vi "test_ccd_parseImageData.vi"(8 "error in (no error)":errorcluster) -> (0 "error out":errorcluster)   [LabVIEW 2023, in "horiba.test.lvlib"]
uses:
  horiba.test.lvlib
  Classes/CCD/acquisitionData.ctl
  Classes/CCD/CCDImageData.ctl
  <vilib>/addons/_JKI Toolkits/Caraya/classes/Assert/Assert Not Error.vi
  <vilib>/addons/_JKI Toolkits/Caraya/classes/Assert/Assert Equal Value and Type_Variant.vi
  <vilib>/addons/_JKI Toolkits/Caraya/classes/Test/Test.lvclass
  <vilib>/addons/_JKI Toolkits/Caraya/classes/Assert/Assert.lvclass
  Classes/CCD/CCD.lvclass
panel:
  # "Connector Pane"
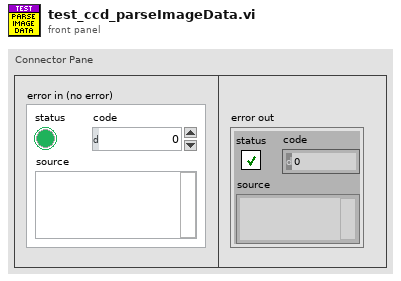
[diagram p1: front panel]
types:
  T1 = typedef "horiba.lvlib/CCD.lvclass/acquisitionData.ctl" = cluster{"acqIndex":i32, "ROIs":T2[]}
  T2 = typedef "horiba.lvlib/CCD.lvclass/CCDImageData.ctl" = cluster{"roiIndex":i32, "xBinning":i32, "xOrigin":i32, "xSize":i32, "yBinning":i32, "yOrigin":i32, "ySize":i32, "xAxis":dbl[], "Data":dbl[][]}
  T3 = typedef "acquisitionData.ctl" = cluster{"acqIndex":i32, "ROIs":T2[]}
diagram:
  n1 = call <vilib>:"Define Test.vi"("error in (no error)"="error in (no error)") -> ("error out"=w7:errorcluster)  [unwired: 9 in, 1 out]
  "error out" <- w7
  n2 = call "parseImageData.vi"("results-JSON string"="{\"acquisition\":[{\"acqIndex\":1,\"roi\":[{\"roiIndex\":1,\"xBinning\":1,\"xOrigin\":0,\"xSize\":1024,\"xyData\":[[0,608],[1,606],[2,607],[3,606],[4,605],[5,606],[6,604],[7,607],[8,605],[9,605],[10,606],[11,606],[12,604],[13,604],[14,604],[15,607],[16,606],[17,606],[18,604],[19,606],[20,607],[21,607],[22,606],[23,608],[24,606],[25,605],[26,607],[27,605],[28,607],[29,607],[30,604],[31,606],[32,608],[33,605],[34,606],[35,607],[36,603],[37,605],[38,605],[39,606],[40,605],[41,606],[42,605],[43,607],[44,606],[45,607],[46,605],[47,605],[48,607],[49,606],[50,606],[51,606],[52,605],[53,607],[54,607],[55,604],[56,607],[57,608],[58,607],[59,608],[60,606],[61,605],[62,608],[63,606],[64,605],[65,606],[66,604],[67,607],[68,607],[69,607],[70,611],[71,608],[72,606],[73,608],[74,607],[75,603],[76,604],[77,607],[78,604],[79,606],[80,606],[81,608],[82,603],[83,604],[84,607],[85,605],[86,605],[87,605],[88,607],[89,605],[90,606],[91,606],[92,608],[93,605],[94,606],[95,605],[96,609],[97,606],[98,609],[99,606],[100,605],[101,605],[102,607],[103,605],[104,606],[105,605],[106,607],[107,605],[108,607],[109,609],[110,604],[111,605],[112,605],[113,606],[114,606],[115,604],[116,606],[117,608],[118,606],[119,606],[120,603],[121,604],[122,607],[123,605],[124,604],[125,604],[126,608],[127,603],[128,605],[129,607],[130,605],[131,608],[132,604],[133,605],[134,602],[135,605],[136,606],[137,607],[138,604],[139,602],[140,604],[141,607],[142,606],[143,607],[144,607],[145,605],[146,606],[147,606],[148,607],[149,606],[150,603],[151,604],[152,604],[153,605],[154,607],[155,606],[156,605],[157,606],[158,608],[159,607],[160,605],[161,606],[162,604],[163,605],[164,606],[165,610],[166,607],[167,605],[168,608],[169,607],[170,606],[171,606],[172,606],[173,606],[174,604],[175,607],[176,606],[177,605],[178,606],[179,606],[180,605],[181,608],[182,605],[183,604],[184,607],[185,605],[186,609],[187,606],[188,603],[189,604],[190,607],[191,603],[192,608],[193,606],[194,607],[195,608],[196,607],[197,607],[198,606],[199,607],[200,607],[201,606],[202,605],[203,606],[204,606],[205,606],[206,604],[207,605],[208,607],[209,609],[210,608],[211,606],[212,608],[213,605],[214,608],[215,606],[216,606],[217,607],[218,605],[219,603],[220,606],[221,604],[222,606],[223,606],[224,607],[225,605],[226,607],[227,607],[228,609],[229,604],[230,607],[231,605],[232,602],[233,607],[234,605],[235,607],[236,608],[237,605],[238,606],[239,609],[240,605],[241,607],[242,605],[243,605],[244,608],[245,606],[246,609],[247,605],[248,604],[249,606],[250,606],[251,608],[252,605],[253,607],[254,605],[255,605],[256,606],[257,607],[258,606],[259,607],[260,605],[261,608],[262,608],[263,606],[264,606],[265,606],[266,608],[267,608],[268,607],[269,608],[270,606],[271,606],[272,606],[273,606],[274,606],[275,607],[276,606],[277,606],[278,603],[279,608],[280,607],[281,605],[282,606],[283,607],[284,607],[285,605],[286,606],[287,606],[288,607],[289,605],[290,607],[291,604],[292,605],[293,608],[294,608],[295,607],[296,607],[297,608],[298,607],[299,607],[300,608],[301,605],[302,607],[303,604],[304,605],[305,606],[306,609],[307,605],[308,607],[309,607],[310,606],[311,606],[312,606],[313,605],[314,606],[315,607],[316,606],[317,608],[318,606],[319,605],[320,611],[321,608],[322,607],[323,604],[324,608],[325,606],[326,611],[327,606],[328,608],[329,606],[330,608],[331,608],[332,607],[333,608],[334,605],[335,607],[336,608],[337,607],[338,608],[339,609],[340,608],[341,605],[342,604],[343,604],[344,606],[345,605],[346,605],[347,608],[348,610],[349,606],[350,609],[351,605],[352,609],[353,605],[354,607],[355,608],[356,608],[357,607],[358,605],[359,609],[360,608],[361,607],[362,604],[363,605],[364,609],[365,607],[366,607],[367,609],[368,608],[369,606],[370,607],[371,609],[372,608],[373,608],[374,605],[375,607],[376,607],[377,607],[378,605],[379,605],[380,605],[381,607],[382,607],[383,607],[384,607],[385,604],[386,608],[387,605],[388,609],[389,609],[390,606],[391,607],[392,607],[393,609],[394,607],[395,606],[396,605],[397,610],[398,608],[399,603],[400,607],[401,608],[402,606],[403,604],[404,609],[405,608],[406,605],[407,609],[408,604],[409,607],[410,604],[411,608],[412,608],[413,607],[414,605],[415,606],[416,606],[417,607],[418,605],[419,606],[420,608],[421,609],[422,605],[423,608],[424,606],[425,605],[426,607],[427,606],[428,606],[429,606],[430,607],[431,606],[432,606],[433,605],[434,605],[435,607],[436,606],[437,606],[438,607],[439,605],[440,606],[441,606],[442,608],[443,605],[444,607],[445,604],[446,608],[447,606],[448,607],[449,605],[450,605],[451,606],[452,609],[453,607],[454,608],[455,605],[456,608],[457,605],[458,604],[459,607],[460,606],[461,606],[462,607],[463,608],[464,607],[465,606],[466,606],[467,605],[468,605],[469,606],[470,608],[471,607],[472,606],[473,606],[474,605],[475,606],[476,608],[477,607],[478,607],[479,608],[480,605],[481,606],[482,606],[483,604],[484,605],[485,606],[486,605],[487,605],[488,605],[489,607],[490,607],[491,603],[492,606],[493,606],[494,606],[495,608],[496,606],[497,605],[498,606],[499,608],[500,607],[501,607],[502,609],[503,607],[504,606],[505,605],[506,609],[507,606],[508,606],[509,607],[510,607],[511,607],[512,607],[513,606],[514,610],[515,607],[516,609],[517,606],[518,607],[519,608],[520,604],[521,608],[522,605],[523,607],[524,607],[525,606],[526,607],[527,605],[528,605],[529,609],[530,608],[531,607],[532,607],[533,606],[534,607],[535,606],[536,605],[537,608],[538,606],[539,606],[540,606],[541,608],[542,606],[543,606],[544,605],[545,607],[546,608],[547,608],[548,608],[549,606],[550,606],[551,605],[552,607],[553,606],[554,605],[555,605],[556,607],[557,605],[558,608],[559,603],[560,609],[561,608],[562,606],[563,609],[564,603],[565,606],[566,608],[567,605],[568,605],[569,607],[570,606],[571,609],[572,606],[573,607],[574,606],[575,606],[576,609],[577,605],[578,606],[579,603],[580,606],[581,608],[582,608],[583,608],[584,606],[585,602],[586,605],[587,605],[588,605],[589,606],[590,608],[591,604],[592,610],[593,606],[594,605],[595,605],[596,609],[597,609],[598,608],[599,606],[600,606],[601,605],[602,605],[603,608],[604,604],[605,608],[606,609],[607,605],[608,611],[609,606],[610,607],[611,606],[612,608],[613,605],[614,605],[615,605],[616,604],[617,605],[618,605],[619,609],[620,609],[621,605],[622,606],[623,605],[624,606],[625,607],[626,607],[627,606],[628,604],[629,605],[630,607],[631,607],[632,607],[633,607],[634,607],[635,605],[636,605],[637,606],[638,607],[639,606],[640,606],[641,607],[642,607],[643,605],[644,604],[645,604],[646,605],[647,606],[648,608],[649,607],[650,606],[651,606],[652,605],[653,606],[654,605],[655,607],[656,606],[657,606],[658,606],[659,608],[660,608],[661,606],[662,607],[663,604],[664,604],[665,606],[666,604],[667,607],[668,605],[669,604],[670,605],[671,605],[672,607],[673,609],[674,604],[675,604],[676,607],[677,606],[678,607],[679,605],[680,607],[681,607],[682,604],[683,606],[684,609],[685,604],[686,608],[687,608],[688,606],[689,607],[690,606],[691,606],[692,608],[693,605],[694,604],[695,606],[696,606],[697,605],[698,602],[699,608],[700,609],[701,605],[702,606],[703,603],[704,605],[705,606],[706,606],[707,605],[708,607],[709,606],[710,607],[711,607],[712,610],[713,607],[714,606],[715,609],[716,605],[717,605],[718,605],[719,605],[720,607],[721,605],[722,606],[723,605],[724,605],[725,608],[726,607],[727,609],[728,605],[729,606],[730,604],[731,604],[732,607],[733,604],[734,605],[735,604],[736,607],[737,609],[738,607],[739,606],[740,604],[741,608],[742,604],[743,604],[744,606],[745,608],[746,606],[747,607],[748,605],[749,603],[750,606],[751,605],[752,606],[753,605],[754,606],[755,605],[756,605],[757,608],[758,607],[759,607],[760,606],[761,607],[762,605],[763,608],[764,607],[765,607],[766,606],[767,605],[768,607],[769,607],[770,605],[771,605],[772,604],[773,607],[774,607],[775,607],[776,604],[777,604],[778,608],[779,603],[780,605],[781,606],[782,606],[783,607],[784,607],[785,605],[786,607],[787,603],[788,604],[789,607],[790,607],[791,609],[792,606],[793,607],[794,607],[795,608],[796,605],[797,606],[798,608],[799,610],[800,606],[801,607],[802,608],[803,606],[804,607],[805,603],[806,607],[807,608],[808,605],[809,608],[810,606],[811,608],[812,607],[813,605],[814,607],[815,606],[816,609],[817,609],[818,607],[819,607],[820,609],[821,611],[822,606],[823,606],[824,606],[825,607],[826,605],[827,608],[828,605],[829,605],[830,608],[831,607],[832,607],[833,606],[834,605],[835,606],[836,603],[837,606],[838,607],[839,608],[840,605],[841,607],[842,606],[843,606],[844,606],[845,609],[846,605],[847,605],[848,608],[849,605],[850,606],[851,605],[852,604],[853,606],[854,609],[855,606],[856,607],[857,608],[858,607],[859,607],[860,606],[861,606],[862,604],[863,607],[864,607],[865,605],[866,602],[867,606],[868,606],[869,609],[870,605],[871,607],[872,608],[873,606],[874,605],[875,605],[876,605],[877,608],[878,608],[879,606],[880,607],[881,605],[882,604],[883,605],[884,606],[885,605],[886,608],[887,605],[888,607],[889,605],[890,605],[891,609],[892,604],[893,605],[894,607],[895,606],[896,607],[897,608],[898,604],[899,604],[900,607],[901,608],[902,606],[903,606],[904,608],[905,604],[906,604],[907,608],[908,607],[909,606],[910,608],[911,605],[912,604],[913,604],[914,607],[915,605],[916,605],[917,602],[918,607],[919,604],[920,604],[921,605],[922,606],[923,607],[924,608],[925,605],[926,608],[927,608],[928,608],[929,606],[930,605],[931,605],[932,607],[933,607],[934,606],[935,605],[936,605],[937,610],[938,603],[939,606],[940,605],[941,606],[942,604],[943,607],[944,604],[945,610],[946,606],[947,606],[948,607],[949,607],[950,608],[951,607],[952,603],[953,606],[954,606],[955,605],[956,606],[957,604],[958,605],[959,605],[960,605],[961,607],[962,607],[963,605],[964,605],[965,606],[966,604],[967,606],[968,607],[969,605],[970,606],[971,603],[972,605],[973,608],[974,606],[975,606],[976,606],[977,608],[978,613],[979,607],[980,605],[981,606],[982,606],[983,606],[984,605],[985,605],[986,609],[987,608],[988,603],[989,605],[990,606],[991,607],[992,606],[993,604],[994,608],[995,607],[996,605],[997,609],[998,606],[999,605],[1000,606],[1001,606],[1002,605],[1003,604],[1004,606],[1005,605],[1006,606],[1007,606],[1008,607],[1009,605],[1010,604],[1011,605],[1012,607],[1013,605],[1014,604],[1015,607],[1016,606],[1017,607],[1018,603],[1019,607],[1020,605],[1021,607],[1022,607],[1023,605]],\"yBinning\":256,\"yOrigin\":0,\"ySize\":256}]}],\"timestamp\":\"2024.11.18 16:05:52.708\"}") -> ("error out"=w2:errorcluster, "Aquisitions"=w4:T3[])  [unwired: 9 in]
  n3 = call-poly <vilib>:"Assert.vi"("Label"="parse spectral return from ICL" ("Label (VI Title)"), "error in (no error)"=w7, "Y"=T1[] [{"acqIndex"=1, "ROIs"=[{"roiIndex"=1, "xBinning"=1, "xOrigin"=0, "xSize"=1024, "yBinning"=256, "yOrigin"=0, "ySize"=256, "xAxis"=array[1024 elements], "Data"=array1x1024[1024 elements]}]}] ("Aquisitions"), "X"=w4) -> ()  [unwired: 6 in, 2 out]
  n4 = call-poly <vilib>:"Assert.vi"("Label"="No error after parsing spectrum", "Not Error?"=w2) -> ()  [unwired: 8 in, 2 out]
